vi "Status Keyprotect.vi"(8 "error in (no error)":errorcluster, 10 "Address (0)":i32, 11 "VISA resource name":refnum<visa-resource-name>) -> (0 "error out":errorcluster, 2 "Keyprotection":bool, 3 "VISA resource name out":refnum<visa-resource-name>)   [LabVIEW 2021, in "Environment Chamber.lvlib" / "Climatic Chamber.lvlib"]
doc: "<b>Key protection monitor</B>\n\nReturns the key protection state."
uses:
  Climatic Chamber.lvlib
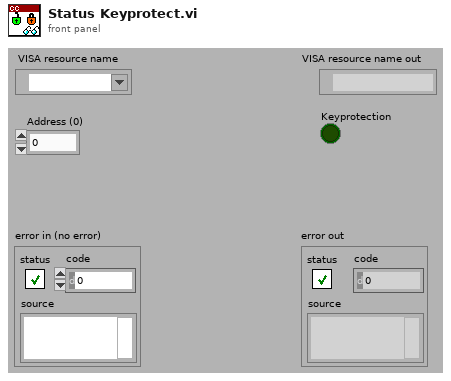
[diagram p1: front panel]
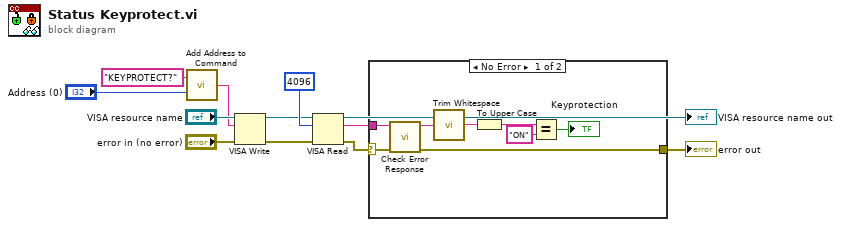
[diagram p0: block diagram]
diagram:
  n1 = call "Add Address to Command.vi"("Address (0)"="Address (0)", "Command"="KEYPROTECT?") -> ("Command OUT"=w5:string)
  n2 = VISA Write(VISA resource name="VISA resource name", write buffer=w5, error in (no error)="error in (no error)") -> (VISA resource name out=w9:refnum<visa-resource-name>, error out=w8:errorcluster)  [unwired: 1 out]
  n3 = VISA Read(VISA resource name=w9, byte count=u32 4096, error in (no error)=w8) -> (VISA resource name out=→"VISA resource name out":refnum<visa-resource-name>, read buffer=w3:string, error out=w4:errorcluster)  [unwired: 1 out]
  n4 = case shown="No Error" w4 {
    selector: w4 -> [w19 w21]
    tunnel: w3 -> [w20 _]
    tunnel: [w17 w21] -> w2
    frame No Error {
      n5 = call "Check Error Response.vi"("error in (no error)"=w19, "read String"=w20) -> ("error out"=w17:errorcluster, "String out"=w18:string)  [unwired: 7 in, 1 out]
      n6 = call <vilib>:"Trim Whitespace.vi"("string"=w18) -> ("trimmed string"=w16:string)  [unwired: 1 in]
      n7 = To Upper Case(1:w16) -> (0:w15:string)
      n8 = Equal?(x=w15, y="ON") -> (x = y?=→"Keyprotection":bool)
    }
    frame Error {
    }
  }
  "error out" <- w2
